vi "Read_Config.vi"() -> ()   [LabVIEW 2025]
uses:
  D:/LV test/LabVIEWConfigSecurity.dll
  LabVIEWConfigSecurity.dll
panel:
  out "输出簇 2":T1
  out "输出簇":T1
  in  "?":T2
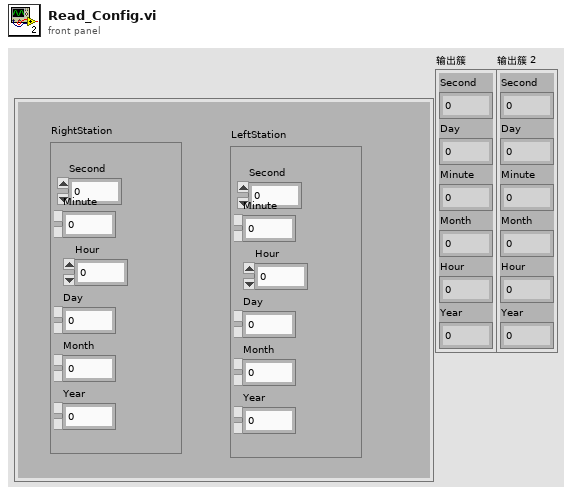
[diagram p1: front panel]
types:
  T1 = cluster{"Second":i32, "Day":i32, "Minute":i32, "Month":i32, "Hour":i32, "Year":i32}
  T2 = cluster{"RightStation":cluster{"Second":i32, "Day":i32, "Minute":i32, "Month":i32, "Hour":i32, "Year":i32}, "LeftStation":cluster{"Second":i32, "Day":i32, "Minute":i32, "Month":i32, "Hour":i32, "Year":i32}}
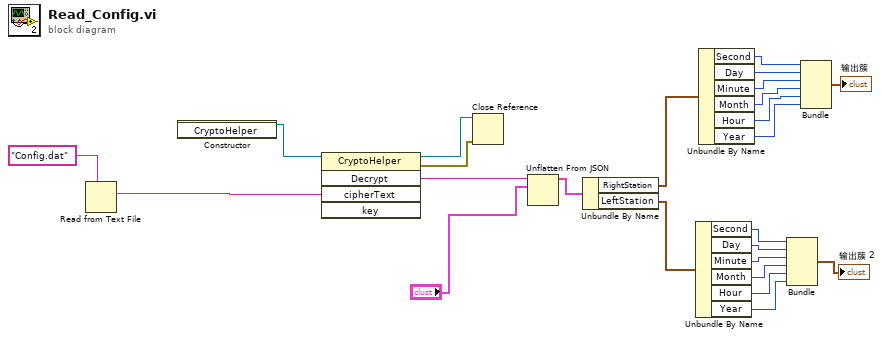
[diagram p0: block diagram]
diagram:
  n1 = Read from Text File(prompt (Open existing file)="Config.dat" ("对话框窗口（打开现有文件）")) -> (text=w22:string)  [unwired: 3 in, 3 out]
  n2 = constructor class="CryptoHelper"() -> (reference out=w23:refnum<k24>)  [unwired: 3 in, 2 out]
  n3 = invoke on="调用节点" class="CryptoHelper" method="Decrypt"(reference=w23, "cipherText"=w22) -> (reference out=w20:refnum<k24>, error out=w19:errorcluster, "Decrypt"=w21:string)  [unwired: 3 in, 2 out]
  n4 = Close Reference(reference=w20, error in (no error)=w19) -> ()  [unwired: 1 out]
  n5 = Unflatten From JSON(JSON string=w21, type and defaults="?") -> (value=w17:T2)  [unwired: 5 in, 1 out]
  n6 = Unbundle By Name(w17) -> ("RightStation"=w16:T1, "LeftStation"=w15:T1)
  n7 = Unbundle By Name(w15) -> ("Second"=w8:i32, "Day"=w7:i32, "Minute"=w6:i32, "Month"=w5:i32, "Hour"=w4:i32, "Year"=w3:i32)
  n8 = Unbundle By Name(w16) -> ("Second"=w14:i32, "Day"=w13:i32, "Minute"=w12:i32, "Month"=w11:i32, "Hour"=w10:i32, "Year"=w9:i32)
  n9 = Bundle("Second"=w8, "Day"=w7, "Minute"=w6, "Month"=w5, "Hour"=w4, "Year"=w3) -> (→"输出簇 2":T1)  [unwired: 1 in]
  n10 = Bundle("Second"=w14, "Day"=w13, "Minute"=w12, "Month"=w11, "Hour"=w10, "Year"=w9) -> (→"输出簇":T1)  [unwired: 1 in]
